vi "SelectMenu4.vi"(0 "XRef":T10, 1 "Tag":T6, 2 "Point":T8, 3 "Click Type":T7, 4 "State In":T1 {"BlockNodeState"."Draw Style" items=["FunctionBlock", "ExpressVI", "Variable", "Elemental I/O", "32x32 Icon", "FunctionBlockCompact"]; "BlockNodeState"."Terminal Data"."Terminal Flags" format="%.0b"}) -> (14 "Reply":T5, 16 "State Out":T1 {"BlockNodeState"."Draw Style" items=["FunctionBlock", "ExpressVI", "Variable", "Elemental I/O", "32x32 Icon", "FunctionBlockCompact"]; "BlockNodeState"."Terminal Data"."Terminal Flags" format="%.0b"})   [LabVIEW 2017, in "NI_Robotics_Create Steering Frame.xnode"]
uses:
  <vilib>/robotics/Steering/Create Steering Frame/NI_Robotics_Create Steering Frame.xnode
  <vilib>/XNodeSupport/XNodeXNodeRef.ctl
  <vilib>/XNodeSupport/XNodeString.ctl
  <vilib>/XNodeSupport/XNodePoint.ctl
  <vilib>/XNodeSupport/XNodeInt.ctl
  <vilib>/XNodeSupport/XNodeClickTypes.ctl
  <vilib>/robotics/Steering/Create Steering Frame/State.ctl
  <vilib>/BlockNodeSupport/BlockNodeState.ctl
  <vilib>/BlockNodeSupport/TerminalData.ctl
  <vilib>/picture/picture.llb/imagedata.ctl
  <vilib>/XNodeSupport/XNodeStringArray.ctl
  <vilib>/XNodeSupport/NI_XNodeSupport.lvlib
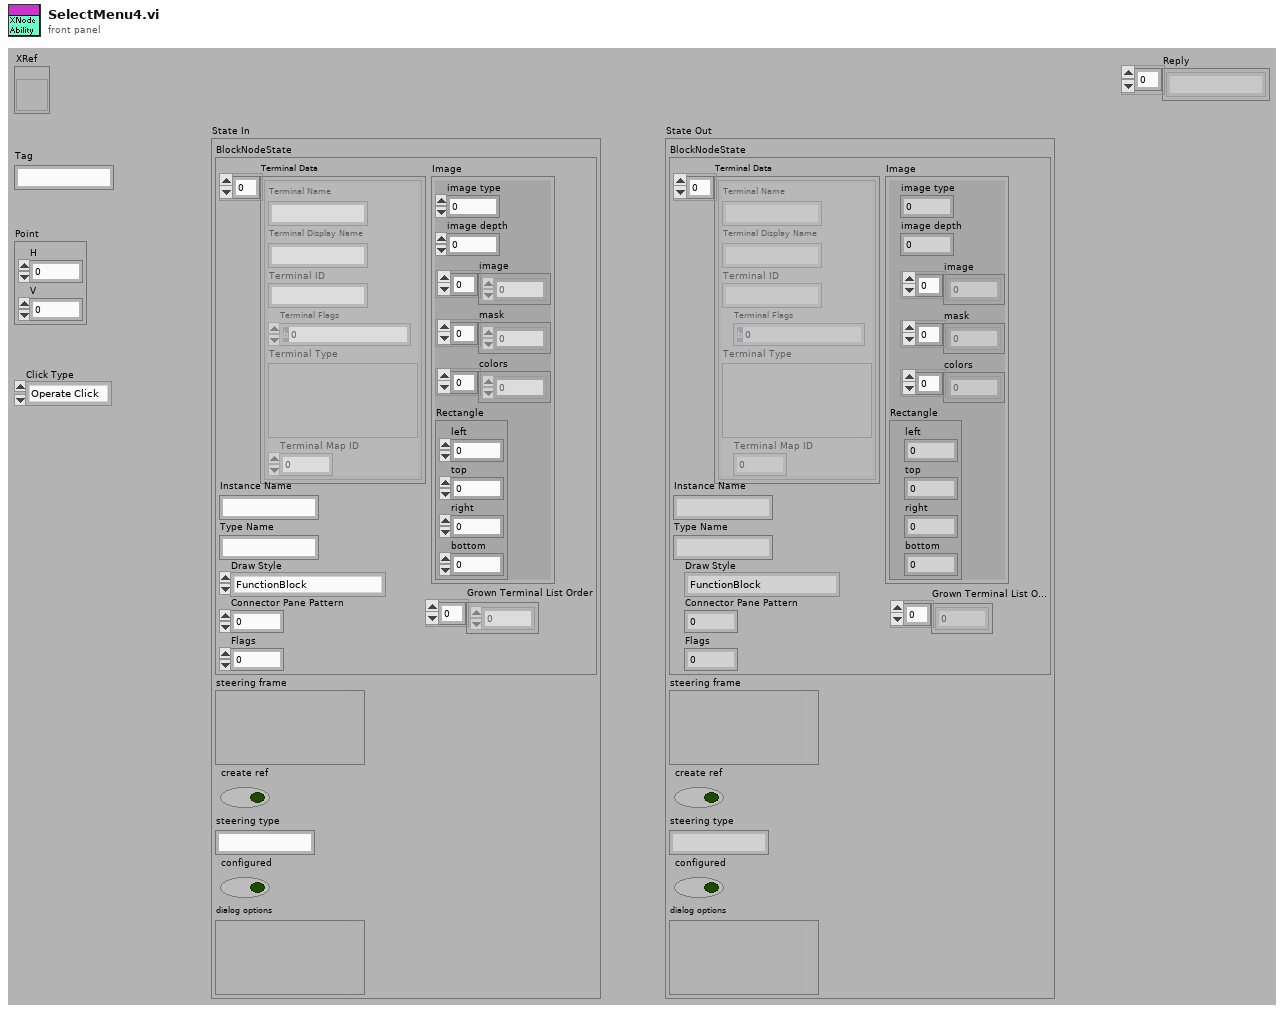
[diagram p1: front panel]
types:
  T1 = typedef "NI_Robotics_Create Steering Frame.xnode/State.ctl" = cluster{"BlockNodeState":T2, "steering frame":variant, "create ref":bool, "steering type":string, "configured":bool, "dialog options":variant}
  T2 = typedef "BlockNodeState.ctl" = cluster{"Terminal Data":T3[], "Instance Name":string, "Type Name":string, "Draw Style":i32, "Connector Pane Pattern":i32, "Flags":i32, "Grown Terminal List Order":i32[], "Image":T4}
  T3 = typedef "TerminalData.ctl" = cluster{"Terminal Name":string, "Terminal Display Name":string, "Terminal ID":string, "Terminal Flags":i32, "Terminal Type":variant, "Terminal Map ID":i32}
  T4 = typedef "imagedata.ctl" = cluster{"image type":i32, "image depth":i32, "image":u8[], "mask":u8[], "colors":u32[], "Rectangle":cluster{"left":i16, "top":i16, "right":i16, "bottom":i16}}
  T5 = typedef "NI_XNodeSupport.lvlib/XNodeStringArray.ctl" = T6[]
  T6 = typedef "NI_XNodeSupport.lvlib/XNodeString.ctl" = string
  T7 = typedef "NI_XNodeSupport.lvlib/XNodeClickTypes.ctl" = enum32{"Operate Click", "Popup Click"}
  T8 = typedef "NI_XNodeSupport.lvlib/XNodePoint.ctl" = cluster{"H":T9, "V":T9}
  T9 = typedef "NI_XNodeSupport.lvlib/XNodeInt.ctl" = i32
  T10 = typedef "NI_XNodeSupport.lvlib/XNodeXNodeRef.ctl" = refnum<vi>
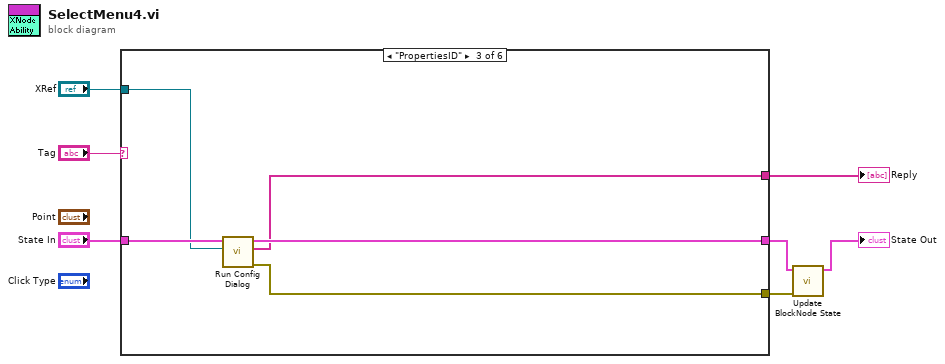
[diagram p0: block diagram]
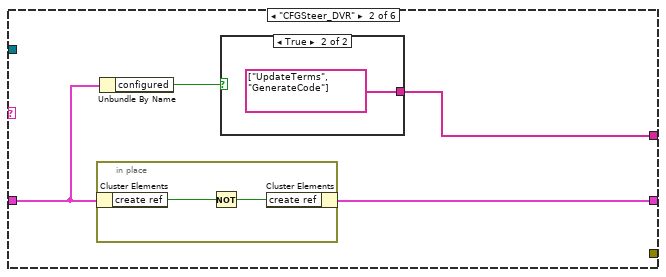
[diagram p3: hidden frame]
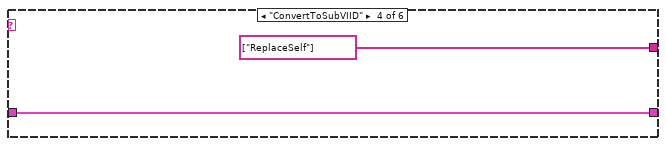
[diagram p5: hidden frame]
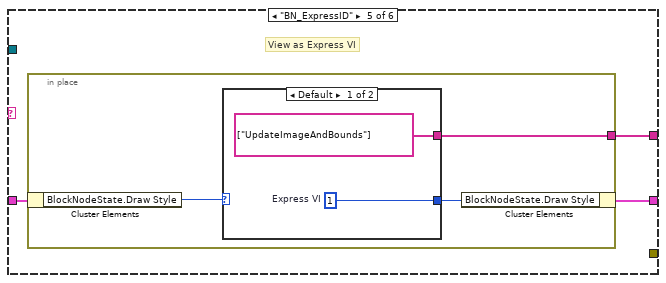
[diagram p6: hidden frame]
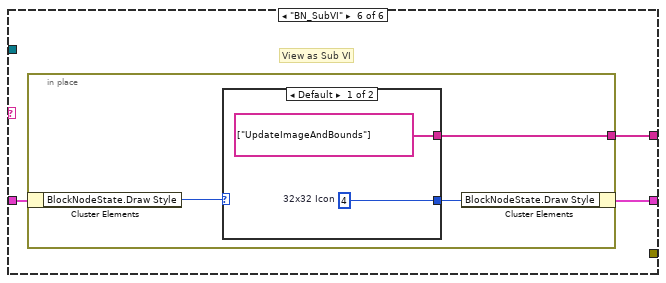
[diagram p8: hidden frame]
diagram:
  n1 = case shown="\"PropertiesID\"" "Tag" {
    tunnel: "State In" -> [w8 w12 w20 w21 w25 w34]
    tunnel: [w8 w11 w19 w21 w24 w33] -> w3
    tunnel: [_ w9 w17 T5 ["ReplaceSelf"] ("Reply") w23 w32] -> w6
    tunnel: [_ _ w18 _ _ _] -> w2
    tunnel: "XRef" -> [_ _ w16 _ _ _]
    frame Default {
    }
    frame "CFGSteer_DVR" {
      n2 = in-place {
        n3 = in-place-cluster #1(w12) -> ("create ref"=w15:bool)
        n4 = Not(x=w15) -> (.not. x?=w14:bool)
        n5 = in-place-cluster #1("create ref"=w14) -> (w11:T1)
      }
      n6 = Unbundle By Name(w12) -> ("configured"=w10:bool)
      n7 = case shown="True" w10 {
        tunnel: [_ T5 ["UpdateTerms", "GenerateCode"] ("Reply")] -> w9
        frame False {
        }
        frame True {
        }
      }
    }
    frame "PropertiesID" {
      n8 = call <vilib>:"Run Config Dialog.vi"("XRef"=w16, "State In"=w20) -> ("error out"=w18:errorcluster, "Reply"=w17:T5, "State Out"=w19:T1)  [unwired: 7 in]
    }
    frame "ConvertToSubVIID" {
    }
    frame "BN_ExpressID" {
      # "View as Express VI"
      n9 = in-place {
        in-place-border: [w28] -> w23
        n10 = in-place-cluster #2(w25) -> ("BlockNodeState.Draw Style"=w27:i32)
        n11 = case shown="Default" w27 {
          selector: w27 -> [_ w31]
          tunnel: [T5 ["UpdateImageAndBounds"] ("Reply") _] -> w28
          tunnel: [w29 w31] -> w26
          frame Default {
            w29 = 1  # Express VI
          }
          frame 1 {
            # "Do nothing if it is already viewed as an Express VI."
          }
        }
        n12 = in-place-cluster #2("BlockNodeState.Draw Style"=w26) -> (w24:T1)
      }
    }
    frame "BN_SubVI" {
      # "View as Sub VI"
      n13 = in-place {
        in-place-border: [w37] -> w32
        n14 = in-place-cluster #3(w34) -> ("BlockNodeState.Draw Style"=w36:i32)
        n15 = case shown="Default" w36 {
          selector: w36 -> [_ w40]
          tunnel: [T5 ["UpdateImageAndBounds"] ("Reply") _] -> w37
          tunnel: [w38 w40] -> w35
          frame Default {
            w38 = 4  # 32x32 Icon
          }
          frame 4 {
            # "Do nothing if it is already viewed as a Sub VI."
          }
        }
        n16 = in-place-cluster #3("BlockNodeState.Draw Style"=w35) -> (w33:T1)
      }
    }
  }
  "Reply" <- w6
  n17 = call <vilib>:"Update BlockNode State.vi"("error in (no error)"=w2, "State in"=w3) -> ("State out"=→"State Out":T1)  [unwired: 8 in, 1 out]
